vi "IHM_callback_step.vi"(4 "entrée d'erreur (pas d'erreur)":errorcluster, 5 "next step no error In":T1, 6 "New lines In":string, 7 "CONSOLE ref In":refnum<vi>) -> (0 "sortie d'erreur":errorcluster, 1 "Next step Out":T1, 3 "CONSOLE ref Out":refnum<vi>)   [LabVIEW 2009]
uses:
  Commands/IHM_cases.ctl
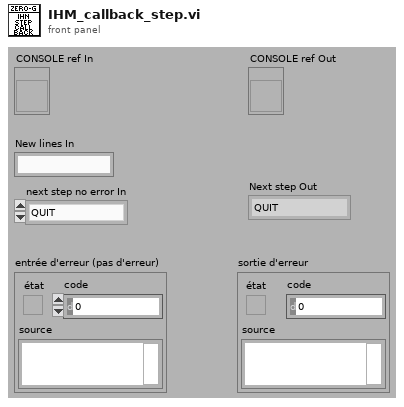
[diagram p1: front panel]
types:
  T1 = typedef "IHM_cases.ctl" = enum16{"QUIT", "INIT IHM", "LOAD CONFIGURATION FILE", "INIT INSTRU", "IHM PROCESS", "CLOSE INSTRU"}
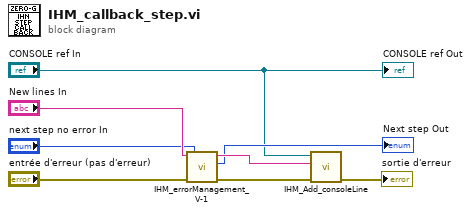
[diagram p0: block diagram]
diagram:
  n1 = call "IHM_errorManagement_V-1.vi"("error out"="entrée d'erreur (pas d'erreur)", "Cas no error"="next step no error In", "No error Line"="New lines In") -> ("entrée d'erreur (pas d'erreur)"=w6:errorcluster, "Cas IHM"=→"Next step Out":T1, "New line Out"=w4:string)  [unwired: 2 in]
  n2 = call "IHM_Add_consoleLine.vi"("entrée d'erreur (pas d'erreur)"=w6, "New line In"=w4, "CONSOLE Ref In"="CONSOLE ref In") -> ("sortie d'erreur"=→"sortie d'erreur":errorcluster)  [unwired: 4 in]
  "CONSOLE ref Out" <- "CONSOLE ref In"
